vi "ToDB.vi"   [LabVIEW 2014]
uses:
  Begin/Global Variables.vi
  <vilib>/Rock Robotics/Network Tables/SD Write Number.vi
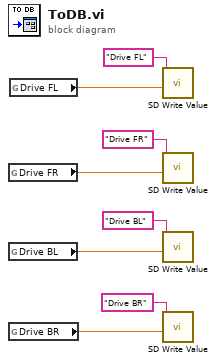
[diagram p0: block diagram]
diagram:
  n1 = global read "Global Variables.vi" "Drive FR"() -> (w7:dbl)
  n2 = global read "Global Variables.vi" "Drive BL"() -> (w6:dbl)
  n3 = global read "Global Variables.vi" "Drive BR"() -> (w5:dbl)
  n4 = global read "Global Variables.vi" "Drive FL"() -> (w8:dbl)
  n5 = call-poly <vilib>:"SD Write Value.vi"("Numeric"=w8, "Name"="Drive FL") -> ()  [unwired: 8 in, 2 out]
  n6 = call-poly <vilib>:"SD Write Value.vi"("Numeric"=w7, "Name"="Drive FR") -> ()  [unwired: 8 in, 2 out]
  n7 = call-poly <vilib>:"SD Write Value.vi"("Numeric"=w6, "Name"="Drive BL") -> ()  [unwired: 8 in, 2 out]
  n8 = call-poly <vilib>:"SD Write Value.vi"("Numeric"=w5, "Name"="Drive BR") -> ()  [unwired: 8 in, 2 out]
